vi "DrawCross.vi"(6 "color(green)":u32(colorbox)=6618880, 8 "error out 2":errorcluster, 10 "Center":cluster{"X":dbl, "Y":dbl}, 11 "Image In":T1) -> (0 "error out":errorcluster, 3 "Image Out":T1)   [LabVIEW 2015]
uses:
  <vilib>/vision/Image Controls.llb/IMAQ Image.ctl
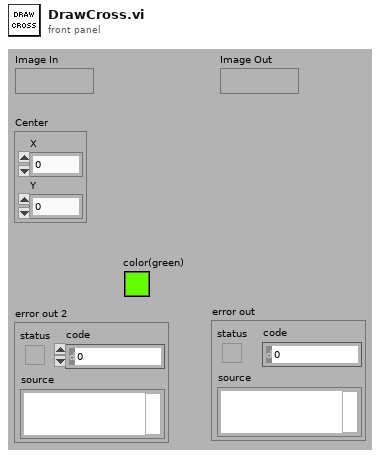
[diagram p1: front panel]
types:
  T1 = typedef "IMAQ Image.ctl" = refnum<image>
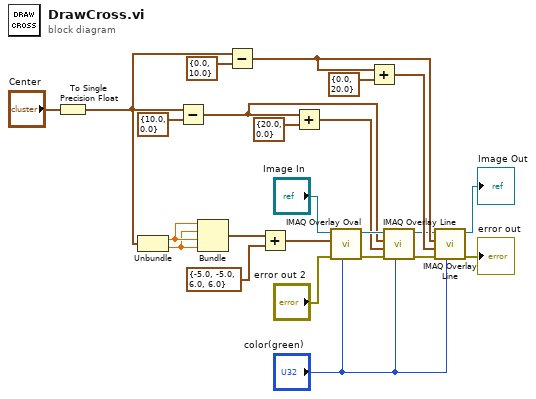
[diagram p0: block diagram]
diagram:
  n1 = To Single Precision Float(number="Center") -> (single precision float=w1:cluster{"X":sgl, "Y":sgl})
  n2 = Unbundle(w1) -> ("X"=w16:sgl, "Y"=w15:sgl)
  n3 = Subtract(x=w1, y=cluster{"x":sgl, "y":sgl} {"x"=10.0, "y"=0.0}) -> (x-y=w10:cluster{sgl, sgl})
  n4 = Bundle("X"=w16, "Y"=w15, "X"=w16, "Y"=w15) -> (w14:cluster{"X":sgl, "Y":sgl, "X":sgl, "Y":sgl})  [unwired: 1 in]
  n5 = Subtract(x=w1, y=cluster{"x":sgl, "y":sgl} {"x"=0.0, "y"=10.0}) -> (x-y=w6:cluster{sgl, sgl})
  n6 = Add(x=w14, y=cluster{"y":sgl, "x":sgl, "y":sgl, "x":sgl} {"y"=-5.0, "x"=-5.0, "y"=6.0, "x"=6.0}) -> (x+y=w12:cluster{sgl, sgl, sgl, sgl})
  n7 = Add(x=w10, y=cluster{"x":sgl, "y":sgl} {"x"=20.0, "y"=0.0}) -> (x+y=w8:cluster{sgl, sgl})
  n8 = call "IMAQ Overlay Oval"("Color"="color(green)", "error in (no error)"="error out 2", "Bounding Rectangle"=w12, "Image"="Image In") -> ("error out"=w17:errorcluster, "Image Out"=w18:T1)  [unwired: 6 in]
  n9 = Add(x=w6, y=cluster{"x":sgl, "y":sgl} {"x"=0.0, "y"=20.0}) -> (x+y=w7:cluster{sgl, sgl})
  n10 = call "IMAQ Overlay Line"("Color"="color(green)", "error in (no error)"=w17, "End Point"=w8, "Start Point"=w10, "Image"=w18) -> ("error out"=w2:errorcluster, "Image Out"=w3:T1)  [unwired: 5 in]
  n11 = call "IMAQ Overlay Line"("Color"="color(green)", "error in (no error)"=w2, "End Point"=w7, "Start Point"=w6, "Image"=w3) -> ("error out"=→"error out":errorcluster, "Image Out"=→"Image Out":T1)  [unwired: 5 in]
